vi "FPGA_SurfaceSingleTouch.vi"() -> ()   [LabVIEW 2014]
uses:
  <vilib>/rvi/Emulation/niFpgaSctlEmulationGetInTimedLoop.vi
  <vilib>/rvi/Emulation/niFpgaProcessEmulError.vi
  <vilib>/rvi/eio/common/nirviEmuTemplateMethod_errors.vi
  <vilib>/rvi/Emulation/niFpgaGetClockAttributes.vi
  <vilib>/rvi/Emulation/niFpgaEmulationReportErrorSimple.vi
  <vilib>/rvi/Memory/Memory_Emulation/nirvimemoryFastEmulation.vi
  <vilib>/rvi/Memory/Memory_Emulation/nirvimemoryEmulation.vi
  <vilib>/rvi/Emulation/niFpgaEmulationIsFPGAContextNoSignature.vi
  <vilib>/rvi/DataTransferAndStorage/Container/Common/niFpgaContainerGetUniqueNameForEmu.vi
  <vilib>/rvi/errors/nirviReportUnexpectedCaseInternalError (U32).vi
  <vilib>/rvi/Emulation/niFpgaCriticalErrorInLSC.vi
  <vilib>/rvi/interface/RandomDataEmulation/niFpgaRandomDataHandleErrors.vi
  <vilib>/eio/EIONode/EIONode.xnode
  <vilib>/rvi/DataTransferAndStorage/Container/XNode/niFpgaContainer.xnode
  <vilib>/rvi/interface/RandomDataEmulation/nirviRandomDataFpgaReadWriteTemplate.vi
panel:
  out "Finished?":bool
  in  "DataRequired?":bool
  out "RTCurr":i16
  out "ZRTPos":i16
  in  "ZWithdrawStepNum":i16
  in  "ZWithdrawStepIndex":i16
  in  "StiffLatency us":i16
  in  "WithdrawLatency us":i16
  in  "GradualWithdraw?":bool
  in  "ThresMultiplier":i16
  in  "stop":bool
  in  "ZDecStepIndex":i16
  in  "MonitorLatency us":i16
  in  "OutputVoltIndex":i16
  in  "DescendCycle":i16
  in  "ZOffset":i16
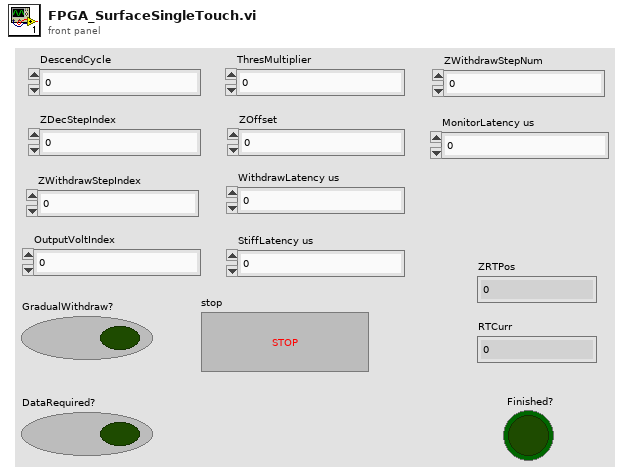
[diagram p1: front panel]
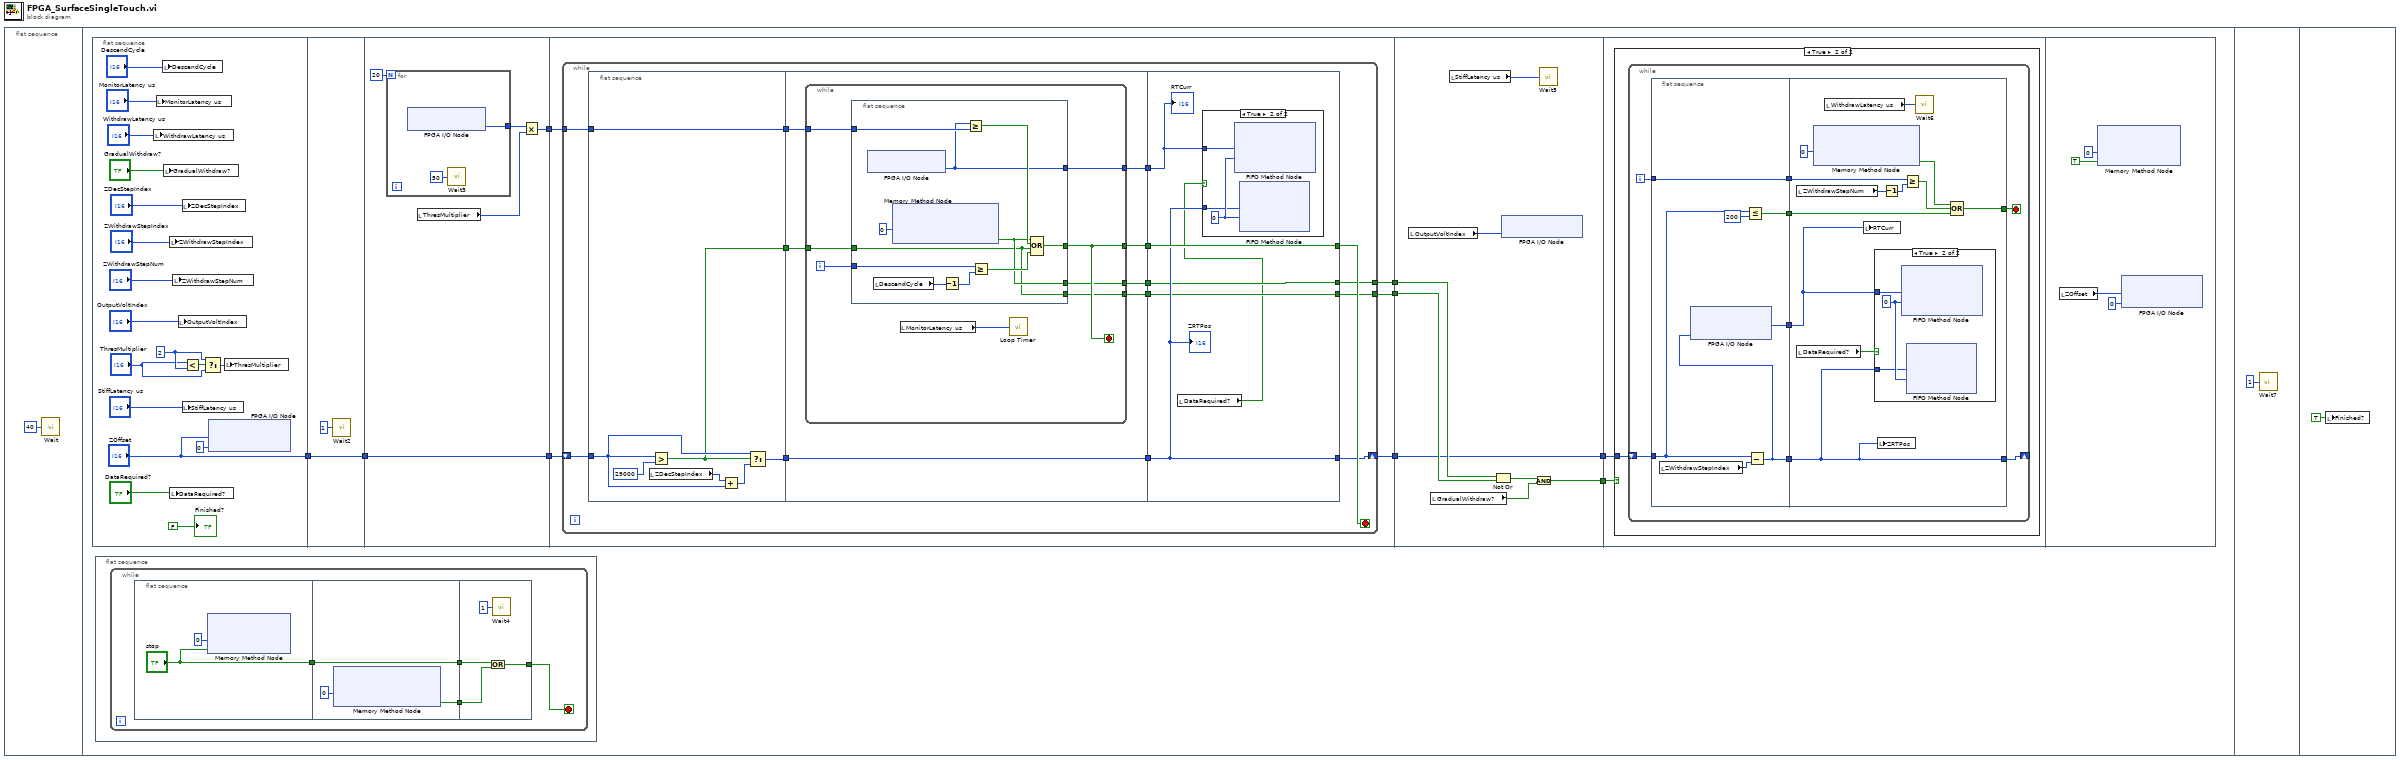
[diagram p0: block diagram]
diagram:
  n1 = flat-sequence {
    frame #0 {
      n2 = call "Wait"("Count(mSec)"=u32 40) -> ()  [unwired: 1 out]
    }
    frame #1 {
      n3 = flat-sequence {
        tunnel: ["ZOffset"] -> w10
        tunnel: [w41] -> w9
        tunnel: w10 -> [w41]
        tunnel: w9 -> [w46]
        tunnel: [w46] -> w8
        tunnel: [w44] -> w7
        tunnel: w8 -> [w54]
        tunnel: w7 -> [w53]
        tunnel: [w52] -> w6
        tunnel: [w51] -> w5
        tunnel: [w50] -> w4
        tunnel: w6 -> [w113]
        tunnel: w5 -> [w117]
        tunnel: w4 -> [w116]
        tunnel: [w113] -> w3
        tunnel: [w112] -> w2
        tunnel: w3 -> [w120]
        tunnel: w2 -> [w119]
        frame #0 {
          w35 = i16 2 ("t")
          n4 = local write "WithdrawLatency us"("WithdrawLatency us") -> ()
          n5 = local write "MonitorLatency us"("MonitorLatency us") -> ()
          n6 = local write "DescendCycle"("DescendCycle") -> ()
          n7 = local write "GradualWithdraw?"("GradualWithdraw?") -> ()
          n8 = local write "ZWithdrawStepIndex"("ZWithdrawStepIndex") -> ()
          n9 = local write "DataRequired?"("DataRequired?") -> ()
          n10 = local write "ZWithdrawStepNum"("ZWithdrawStepNum") -> ()
          n11 = local write "OutputVoltIndex"("OutputVoltIndex") -> ()
          n12 = local write "ZDecStepIndex"("ZDecStepIndex") -> ()
          n13 = local write "StiffLatency us"("StiffLatency us") -> ()
          n14 = Less?(x="ThresMultiplier", y=w35) -> (x < y?=w36:bool)
          n15 = Select(t=w35, s=w36, f="ThresMultiplier") -> (s? t:f=w37:i16)
          n16 = xnode "FPGA I/O Node"("Connector0/AO0"="ZOffset", "Connector0/AO1"=i16 0) -> ()  [unwired: 2 in, 2 out]
          n17 = local write "ThresMultiplier"(w37) -> ()
          "Finished?" <- FALSE ("Finished?")
        }
        frame #1 {
          n18 = call "Wait2"("Count(mSec)"=u32 1) -> ()  [unwired: 1 out]
        }
        frame #2 {
          n19 = for {
            N: 20 -> [_]
            tunnel: [w48] -> w45
            n20 = xnode "FPGA I/O Node"() -> ("Connector0/AI1"=w48:i16)  [unwired: 1 in, 1 out]
            n21 = call "Wait3"("Count(uSec)"=u32 50) -> ()  [unwired: 1 out]
          }
          n22 = local read "ThresMultiplier"() -> (w43:i16)
          n23 = Multiply(x=w45, y=w43) -> (x*y=w44:i16)
        }
        frame #3 {
          n24 = while {
            shift-right: [w59] -> w52
            shift-left: w54 -> [w68]
            tunnel: w53 -> [w67]
            tunnel: [w57] -> w51
            tunnel: [w55] -> w50
            stop <- w63 stop-if-true
            n25 = flat-sequence {
              tunnel: w68 -> [w74]
              tunnel: w67 -> [w69]
              tunnel: [w71] -> w66
              tunnel: [w70] -> w65
              tunnel: [w69] -> w64
              tunnel: w66 -> [w79]
              tunnel: w65 -> [w82]
              tunnel: w64 -> [w81]
              tunnel: [w80] -> w62
              tunnel: [w79] -> w61
              tunnel: [w78] -> w60
              tunnel: [w77] -> w58
              tunnel: [w76] -> w56
              tunnel: [w106] -> w59
              tunnel: [w107] -> w63
              tunnel: w62 -> [w107]
              tunnel: w61 -> [w106]
              tunnel: w60 -> [w103]
              tunnel: [w105] -> w57
              tunnel: w58 -> [w105]
              tunnel: w56 -> [w104]
              tunnel: [w104] -> w55
              frame #0 {
                n26 = local read "ZDecStepIndex"() -> (w72:i16)
                n27 = Greater?(x=w74, y=i16 29000) -> (0:w70:bool)
                n28 = Add(x=w72, y=w74) -> (x+y=w73:i16)
                n29 = Select(t=w74, s=w70, f=w73) -> (s? t:f=w71:i16)
              }
              frame #1 {
                n30 = while {
                  tunnel: w82 -> [w89]
                  tunnel: w81 -> [w88]
                  tunnel: [w86] -> w80
                  tunnel: [w85] -> w78
                  tunnel: [w84] -> w77
                  tunnel: [w83] -> w76
                  i -> [w90]
                  stop <- w86 stop-if-true
                  n31 = flat-sequence {
                    tunnel: w90 -> [w100]
                    tunnel: w89 -> [w93]
                    tunnel: w88 -> [w101]
                    tunnel: [w97] -> w86
                    tunnel: [w95] -> w85
                    tunnel: [w94] -> w84
                    tunnel: [w93] -> w83
                    frame #0 {
                      n32 = xnode "FPGA I/O Node"() -> ("Connector0/AI1"=w95:i16)  [unwired: 1 in, 1 out]
                      n33 = local read "DescendCycle"() -> (w92:i16)
                      n34 = xnode ("Memory Method Node")("Address"=u32 0) -> ("Data"=w94:bool)  [unwired: 1 in, 1 out]
                      n35 = Decrement(x=w92) -> (x-1=w91:i16)
                      n36 = Greater Or Equal?(x=w95, y=w101) -> (x >= y?=w99:bool)
                      n37 = Greater Or Equal?(x=w100, y=w91) -> (x >= y?=w98:bool)
                      n38 = Compound Arithmetic op=OR(w94, w99, w93, w98) -> (w97:bool)
                    }
                  }
                  n39 = local read "MonitorLatency us"() -> (w87:i16)
                  n40 = call "Loop Timer"("Count(Ticks)"=w87) -> ()  [unwired: 1 out]
                }
              }
              frame #2 {
                n41 = local read "DataRequired?"() -> (w102:bool)
                n42 = case shown="True" w102 {
                  tunnel: w106 -> [_ w109]
                  tunnel: w103 -> [_ w108]
                  frame False {
                  }
                  frame True {
                    w110 = 0 ("Timeout")
                    n43 = xnode ("FIFO Method Node")("Element"=w108, "Timeout"=w110) -> ()  [unwired: 1 in, 2 out]
                    n44 = xnode ("FIFO Method Node")("Element"=w109, "Timeout"=w110) -> ()  [unwired: 1 in, 2 out]
                  }
                }
                "ZRTPos" <- w106
                "RTCurr" <- w103
              }
            }
          }
        }
        frame #4 {
          n45 = local read "OutputVoltIndex"() -> (w111:i16)
          n46 = local read "GradualWithdraw?"() -> (w114:bool)
          n47 = local read "StiffLatency us"() -> (w118:i16)
          n48 = Not Or(1:w116, 2:w117) -> (0:w115:bool)
          n49 = xnode "FPGA I/O Node"("Connector0/AO1"=w111) -> ()  [unwired: 1 in, 1 out]
          n50 = And(x=w115, y=w114) -> (x .and. y?=w112:bool)
          n51 = call "Wait5"("Count(uSec)"=w118) -> ()  [unwired: 1 out]
        }
        frame #5 {
          n52 = case shown="True" w119 {
            tunnel: w120 -> [_ w121]
            frame False {
            }
            frame True {
              n53 = while {
                shift-right: [w123] -> _
                shift-left: w121 -> [w129]
                i -> [w126]
                stop <- w124 stop-if-true
                n54 = flat-sequence {
                  tunnel: w129 -> [w135]
                  tunnel: [w131] -> w128
                  tunnel: [w133] -> w127
                  tunnel: w126 -> [w133]
                  tunnel: [w132] -> w125
                  tunnel: [w130] -> w122
                  tunnel: w128 -> [w139]
                  tunnel: w127 -> [w146]
                  tunnel: w125 -> [w141]
                  tunnel: [w140] -> w124
                  tunnel: [w139] -> w123
                  tunnel: w122 -> [w138]
                  frame #0 {
                    n55 = local read "ZWithdrawStepIndex"() -> (w136:i16)
                    n56 = Less Or Equal?(x=w135, y=i16 200) -> (x <= y?=w132:bool)
                    n57 = Subtract(x=w135, y=w136) -> (x-y=w131:i16)
                    n58 = xnode "FPGA I/O Node"("Connector0/AO0"=w131) -> ("Connector0/AI1"=w130:i16)  [unwired: 2 in, 2 out]
                  }
                  frame #1 {
                    n59 = local read "ZWithdrawStepNum"() -> (w145:i16)
                    n60 = local read "DataRequired?"() -> (w137:bool)
                    n61 = xnode ("Memory Method Node")("Address"=u32 0) -> ("Data"=w143:bool)  [unwired: 1 in, 1 out]
                    n62 = local read "WithdrawLatency us"() -> (w148:i16)
                    n63 = local write "RTCurr"(w138) -> ()
                    n64 = case shown="True" w137 {
                      tunnel: w139 -> [_ w150]
                      tunnel: w138 -> [_ w149]
                      frame False {
                      }
                      frame True {
                        w151 = 0 ("Timeout")
                        n65 = xnode ("FIFO Method Node")("Element"=w149, "Timeout"=w151) -> ()  [unwired: 1 in, 2 out]
                        n66 = xnode ("FIFO Method Node")("Element"=w150, "Timeout"=w151) -> ()  [unwired: 1 in, 2 out]
                      }
                    }
                    n67 = local write "ZRTPos"(w139) -> ()
                    n68 = Decrement(x=w145) -> (x-1=w144:i16)
                    n69 = Greater Or Equal?(x=w146, y=w144) -> (x >= y?=w142:bool)
                    n70 = call "Wait6"("Count(uSec)"=w148) -> ()  [unwired: 1 out]
                    n71 = Compound Arithmetic op=OR(w143, w142, w141) -> (w140:bool)
                  }
                }
              }
            }
          }
        }
        frame #6 {
          n72 = local read "ZOffset"() -> (w155:i16)
          n73 = xnode ("Memory Method Node")("Address"=u32 0, "Data"=TRUE) -> ()  [unwired: 1 in, 1 out]
          n74 = xnode "FPGA I/O Node"("Connector0/AO0"=w155, "Connector0/AO1"=i16 0) -> ()  [unwired: 2 in, 2 out]
        }
      }
      n75 = flat-sequence {
        frame #0 {
          n76 = while {
            stop <- w14 stop-if-true
            n77 = flat-sequence {
              tunnel: ["stop"] -> w13
              tunnel: w13 -> [w19]
              tunnel: [w19] -> w12
              tunnel: [w17] -> w11
              tunnel: w12 -> [w21]
              tunnel: [w22] -> w14
              tunnel: w11 -> [w20]
              frame #0 {
                n78 = xnode ("Memory Method Node")("Address"=u32 0, "Data"="stop") -> ()  [unwired: 1 in, 1 out]
              }
              frame #1 {
                n79 = xnode ("Memory Method Node")("Address"=u32 0) -> ("Data"=w17:bool)  [unwired: 1 in, 1 out]
              }
              frame #2 {
                n80 = Or(x=w21, y=w20) -> (x .or. y?=w22:bool)
                n81 = call "Wait4"("Count(mSec)"=u32 1) -> ()  [unwired: 1 out]
              }
            }
          }
        }
      }
    }
    frame #2 {
      n82 = call "Wait7"("Count(mSec)"=u32 1) -> ()  [unwired: 1 out]
    }
    frame #3 {
      n83 = local write "Finished?"(TRUE ("Finished?")) -> ()
    }
  }
